vi "SetValueByItemIndex.vi"(0 "VI Reference In":refnum<vi>, 2 "delimiter (>>)":string=">>", 5 "Control Path":string, 7 "Item Index":i32, 11 "Error In":errorcluster) -> (4 "VI Reference Out":refnum<vi>, 15 "Error Out":errorcluster)   [LabVIEW 2016, in "Drona.lvlib" / "ControlValue.lvlib" / "StimulusListbox.lvlib"]
doc: "Sets value(signaling) for the listbox control whose index is specified. \n\nThe input control name is given as a string , incase of path, use delimiters inbetween the path."
uses:
  StimulusListbox.lvlib
  <vilib>/Utility/error.llb/Error Cluster From Error Code.vi
  <vilib>/ErrorRing/Error Ring.xnode
  Drona.lvlib
  Get/GetControlRef/GetControlRef.lvlib
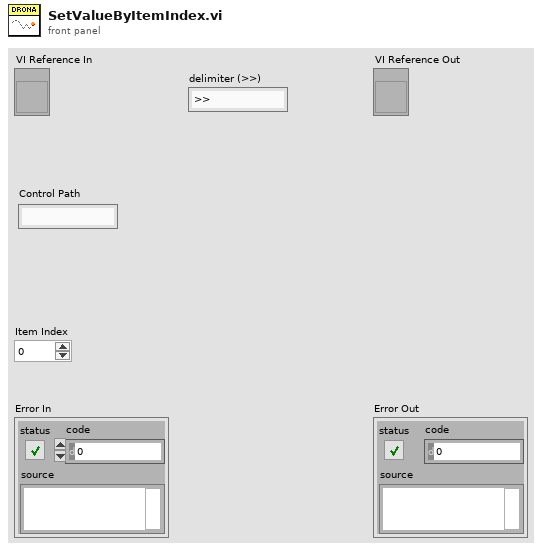
[diagram p1: front panel]
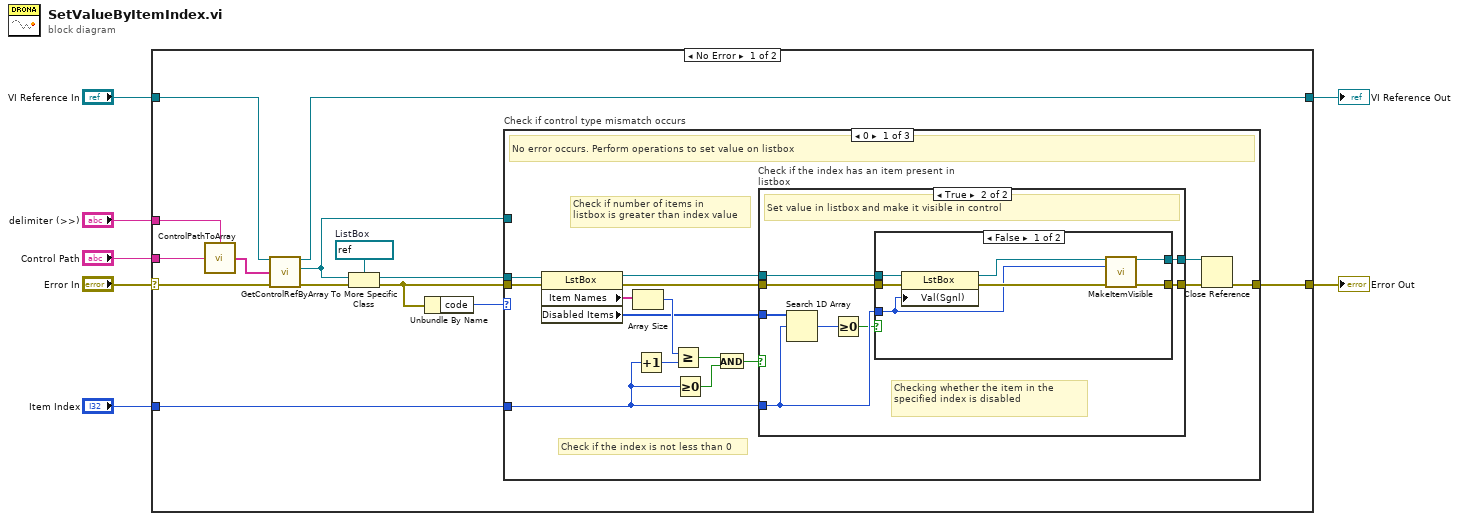
[diagram p0: block diagram]
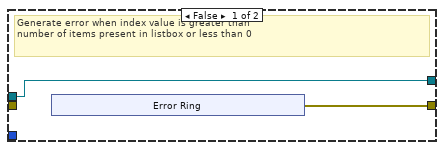
[diagram p2: hidden frame]
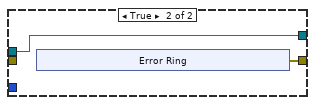
[diagram p3: hidden frame]
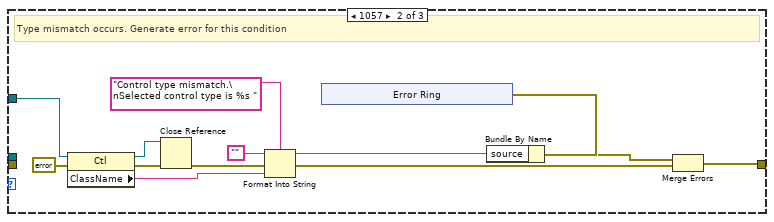
[diagram p4: hidden frame]
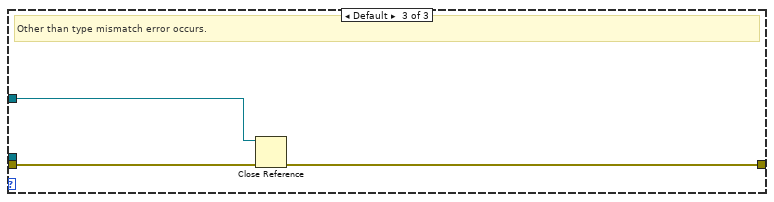
[diagram p5: hidden frame]
diagram:
  n1 = case shown="No Error" "Error In" {
    selector: "Error In" -> [w10 w88]
    tunnel: [w18 w88] -> w6
    tunnel: "VI Reference In" -> [w14 w87]
    tunnel: "Control Path" -> [w20 _]
    tunnel: "Item Index" -> [w16 _]
    tunnel: [w13 w87] -> w2
    tunnel: "delimiter (>>)" -> [w19 _]
    frame No Error {
      w21 = refnum<vi> refnum  # ListBox
      n2 = call "ControlPathToArray.vi"("Control Name"=w20, "delimiter (>>)"=w19) -> ("Control Path"=w15:string[])
      n3 = call "GetControlRefByArray.vi"("VI Reference In"=w14, "Control Path"=w15, "error In"=w10) -> ("VI Reference Out"=w13:refnum<vi>, "Ctl Refnum"=w11:refnum<vi>, "error out"=w12:errorcluster)  [unwired: 10 in]
      n4 = To More Specific Class(target class=w21, reference=w11, error in=w12) -> (specific class reference=w17:refnum<vi>, error out=w9:errorcluster)
      n5 = Unbundle By Name(w9) -> ("code"=w8:i32)
      n6 = case "Check if control type mismatch occurs" shown="0" w8 {
        tunnel: [w36 w68 w85] -> w18
        tunnel: w17 -> [w28 _ _]
        tunnel: w16 -> [w26 _ _]
        tunnel: w11 -> [_ w78 w84]
        tunnel: w9 -> [w35 _ w86]
        frame 0 {
          # "Check if the index is not less than 0"
          # "Check if number of items in \nlistbox is greater than index value"
          # "No error occurs. Perform operations to set value on listbox"
          n7 = property class="LstBox"(reference=w28, error in=w35) -> (reference out=w27:refnum<vi>, error out=w32:errorcluster, "Item Names"=w31:string[], "Disabled Items"=w22:i32[])
          n8 = Array Size(array=w31) -> (size(s)=w30:i32)
          n9 = Increment(x=w26) -> (x+1=w29:i32)
          n10 = Greater Or Equal?(x=w30, y=w29) -> (x >= y?=w25:bool)
          n11 = Greater Or Equal To 0?(x=w26) -> (x >= 0?=w23:bool)
          n12 = And(x=w25, y=w23) -> (x .and. y?=w24:bool)
          n13 = case "Check if the index has an item present in listbox" shown="True" w24 {
            tunnel: [w37 w51] -> w34
            tunnel: [w38 w50] -> w33
            tunnel: w32 -> [_ w49]
            tunnel: w27 -> [w38 w48]
            tunnel: w26 -> [_ w46]
            tunnel: w22 -> [_ w47]
            frame False {
              # "Generate error when index value is greater than \nnumber of items present in listbox or less than 0"
              n14 = xnode "Error Ring"() -> ("error out"=w37:errorcluster)
            }
            frame True {
              # "Checking whether the item in the specified index is disabled"
              # "Set value in listbox and make it visible in control"
              n15 = Search 1D Array(1D array=w47, element=w46) -> (index of element=w44:i32)  [unwired: 1 in]
              n16 = Greater Or Equal To 0?(x=w44) -> (x >= 0?=w45:bool)
              n17 = case shown="False" w45 {
                tunnel: [w58 w59] -> w51
                tunnel: [w57 w60] -> w50
                tunnel: w49 -> [w56 _]
                tunnel: w48 -> [w54 w60]
                tunnel: w46 -> [w53 _]
                frame False {
                  n18 = property class="LstBox"(reference=w54, error in=w56, "Val(Sgnl)"=w53) -> (reference out=w52:refnum<vi>, error out=w55:errorcluster)
                  n19 = call "MakeItemVisible.vi"("ListBox Ref In"=w52, "Item Index"=w53, "Error In"=w55) -> ("ListBox Ref Out"=w57:refnum<vi>, "Error Out"=w58:errorcluster)  [unwired: 11 in]
                }
                frame True {
                  n20 = xnode "Error Ring"() -> ("error out"=w59:errorcluster)
                }
              }
            }
          }
          n21 = Close Reference(reference=w33, error in (no error)=w34) -> (error out=w36:errorcluster)
        }
        frame 1057 {
          # "Type mismatch occurs. Generate error for this condition"
          n22 = property class="Ctl"(reference=w78, error in=errorcluster {"status"=FALSE, "code"=0, "source"=""} ("error out")) -> (reference out=w66:refnum<vi>, error out=w77:errorcluster, "ClassName"=w74:string)
          n23 = Close Reference(reference=w66, error in (no error)=w77) -> (error out=w67:errorcluster)
          n24 = Format Into String(format string="Control type mismatch.\nSelected control type is %s ", initial string="", error in=w67, w74) -> (resulting string=w71:string, error out=w69:errorcluster)
          n25 = xnode "Error Ring"() -> ("error out"=w72:errorcluster)
          n26 = Bundle By Name(cluster=w72, "source"=w71) -> (w70:errorcluster)
          n27 = Merge Errors(w70, w69) -> (w68:errorcluster)
        }
        frame Default {
          # "Other than type mismatch error occurs."
          n28 = Close Reference(reference=w84, error in (no error)=w86) -> (error out=w85:errorcluster)
        }
      }
    }
    frame Error {
    }
  }
  "Error Out" <- w6
  "VI Reference Out" <- w2
